vi "closeDotNetStep.vi"(8 "error in":errorcluster, 11 "NewStep":refnum<k7>) -> (0 "error out":errorcluster)   [LabVIEW 2010]
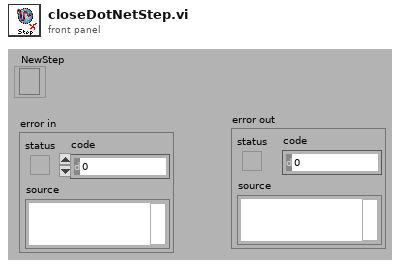
[diagram p1: front panel]
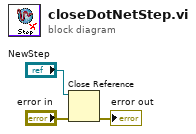
[diagram p0: block diagram]
diagram:
  n1 = Close Reference(reference="NewStep", error in (no error)="error in") -> (error out=→"error out":errorcluster)
